vi "SRXRecoverQuadPosition.vi"(1 "LatestQuadPosition":i32, 2 "AbsoluteOffset":i32, 3 "AbsolutePosition (No Overflow)":i32) -> (0 "RecoveredQuadPosition":i32)   [LabVIEW 2019, in "ArgosLib.lvlib"]
uses:
  d7b33dd1-61b1-4695-a538-69de41910542.vi
  d7b33dd1-61b1-4695-a538-69de41910542.vi/d708faed-a9bf-4cab-ac4e-00044f891ae1.vi
  ArgosLib.lvlib
panel:
  out "LatestAbsolutePosition (withOverflow)":i32
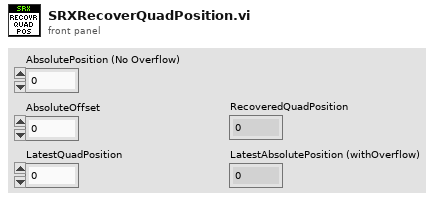
[diagram p1: front panel]
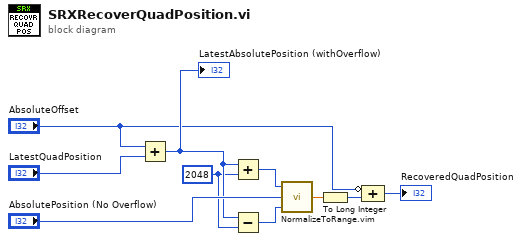
[diagram p0: block diagram]
diagram:
  w7 = 2048 ("y")
  n1 = Add(x="AbsoluteOffset", y="LatestQuadPosition") -> (x+y=w8:i32)
  "LatestAbsolutePosition (withOverflow)" <- w8
  n2 = Add(x=w8, y=w7) -> (x+y=w5:i32)
  n3 = Subtract(x=w8, y=w7) -> (x-y=w6:i32)
  n4 = call "NormalizeToRange.vim"("MinVal"=w6, "x"="AbsolutePosition (No Overflow)", "MaxVal"=w5) -> ("Normalized x"=w4:dbl)
  n5 = To Long Integer(number=w4) -> (32bit integer=w3:i32)
  n6 = Compound Arithmetic op=ADD(invert "AbsoluteOffset", w3) -> (→"RecoveredQuadPosition":i32)
